vi "SubVI_Read_PHD_FromJSON_ver2.4.vi"(6 "Filter SIS by m/z?":bool, 7 "Nominal m/z for SIS hist finding\nComma separated":string, 8 "MAX Event Rate":dbl=0.1 format="%#_13g", 9 "MIN Event Rate":dbl=0.005 format="%#_13g", 10 "file (use dialog)":path) -> (1 "m/z in SIS Hist":dbl[](array[numeric]), 2 "Average SIS from Filtered Data":cluster{dbl[], dbl[]}(graph), 3 "Filtered SIS Hist in mV-ns":dbl[](array[numeric]), 5 "AverageSis":dbl)   [LabVIEW 2018]
uses:
  <vilib>/Analysis/baseanly.llb/Mean (DBL).vi
  <vilib>/Analysis/NI_AALPro.lvlib
  <vilib>/Analysis/NI_AALBase.lvlib
panel:
  out "min value":dbl
  out "SIS median":dbl format="%0.2f"
  out "SIS mean":dbl format="%0.2f"
  out "Original SIS Data":T1
  out "SpectrumCount":dbl
  out "User Filtered SIS Hist":T2(graph)
  out "Nbr Profiles":i32
  out "Profiles":T3(array[cluster])
  out "Original SIS Histogram":cluster{"Intensity":dbl[], "Frequency":dbl[]}(graph)
  out "JSON Text":string
  # "USER Filtering of SIS histogram data"
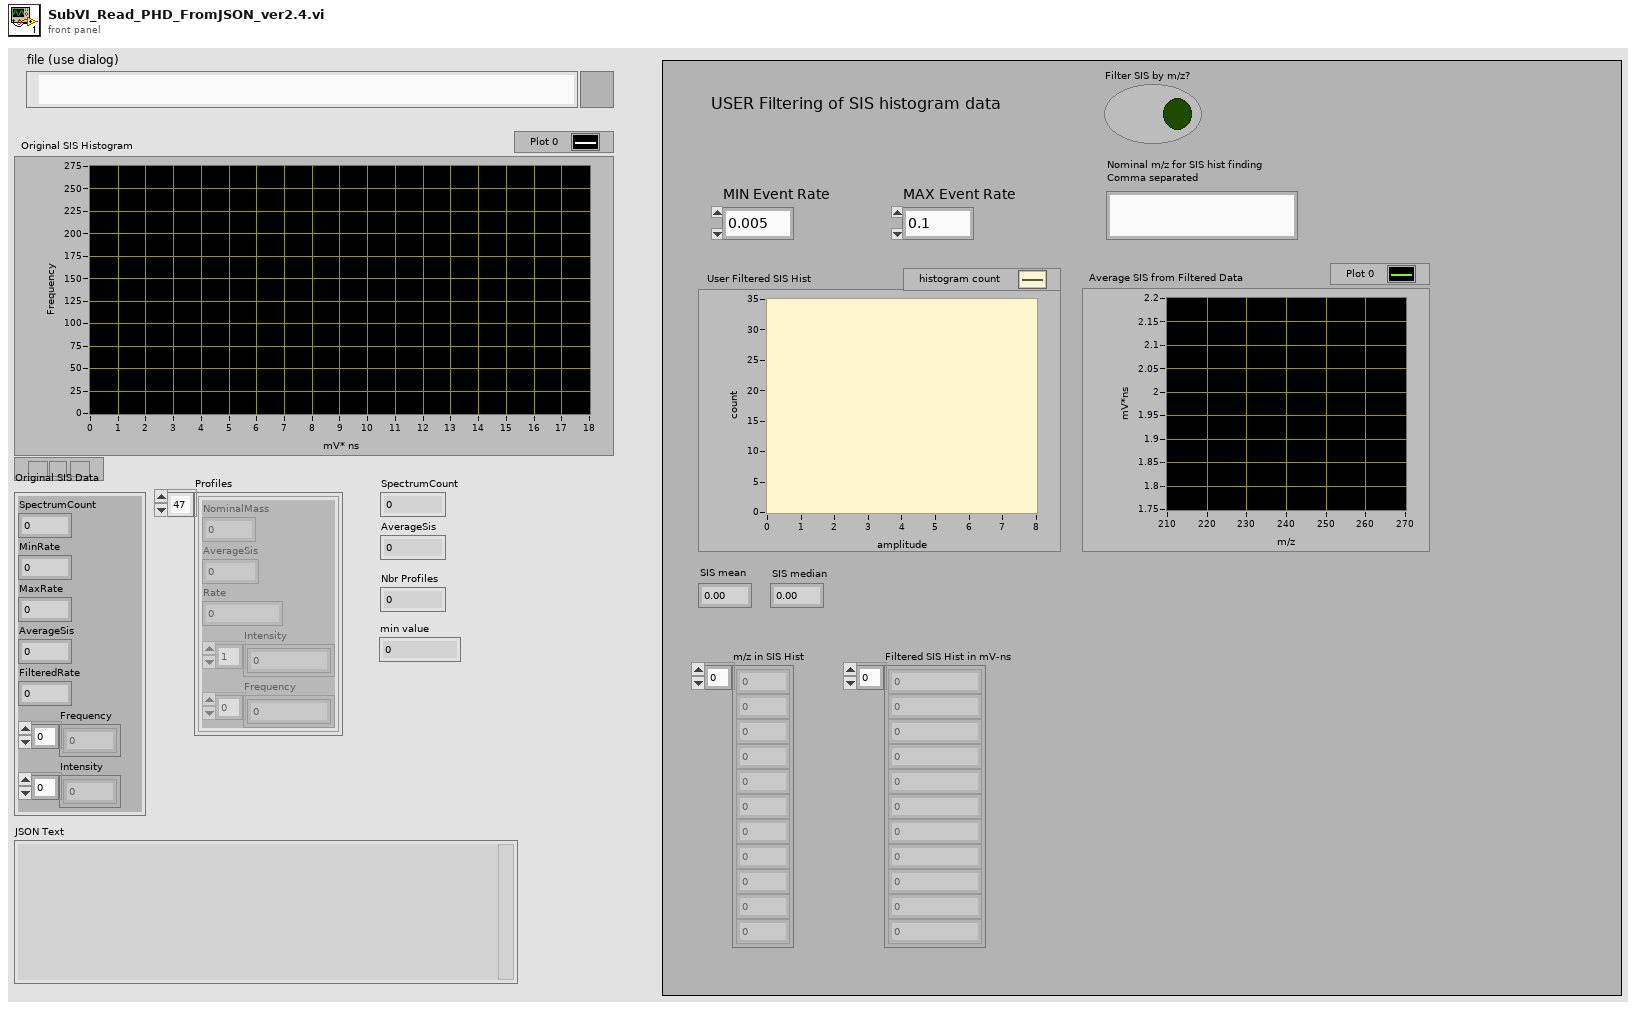
[diagram p1: front panel]
types:
  T1 = cluster{"SpectrumCount":dbl, "MinRate":dbl, "MaxRate":dbl, "AverageSis":dbl, "FilteredRate":dbl, "Frequency":dbl[], "Intensity":dbl[]}
  T2 = cluster{"X Values":dbl[], "Histogram: h(x)":i32[]}
  T3 = cluster{"NominalMass":dbl, "AverageSis":dbl, "Rate":dbl, "Intensity":dbl[], "Frequency":dbl[]}[]
  T4 = cluster{"Profiles":cluster{"NominalMass":dbl, "AverageSis":dbl, "Rate":dbl, "Intensity":dbl[], "Frequency":i32[]}[]}
  T5 = cluster{"NominalMass":dbl, "AverageSis":dbl, "Rate":dbl, "Intensity":dbl[], "Frequency":i32[]}[]
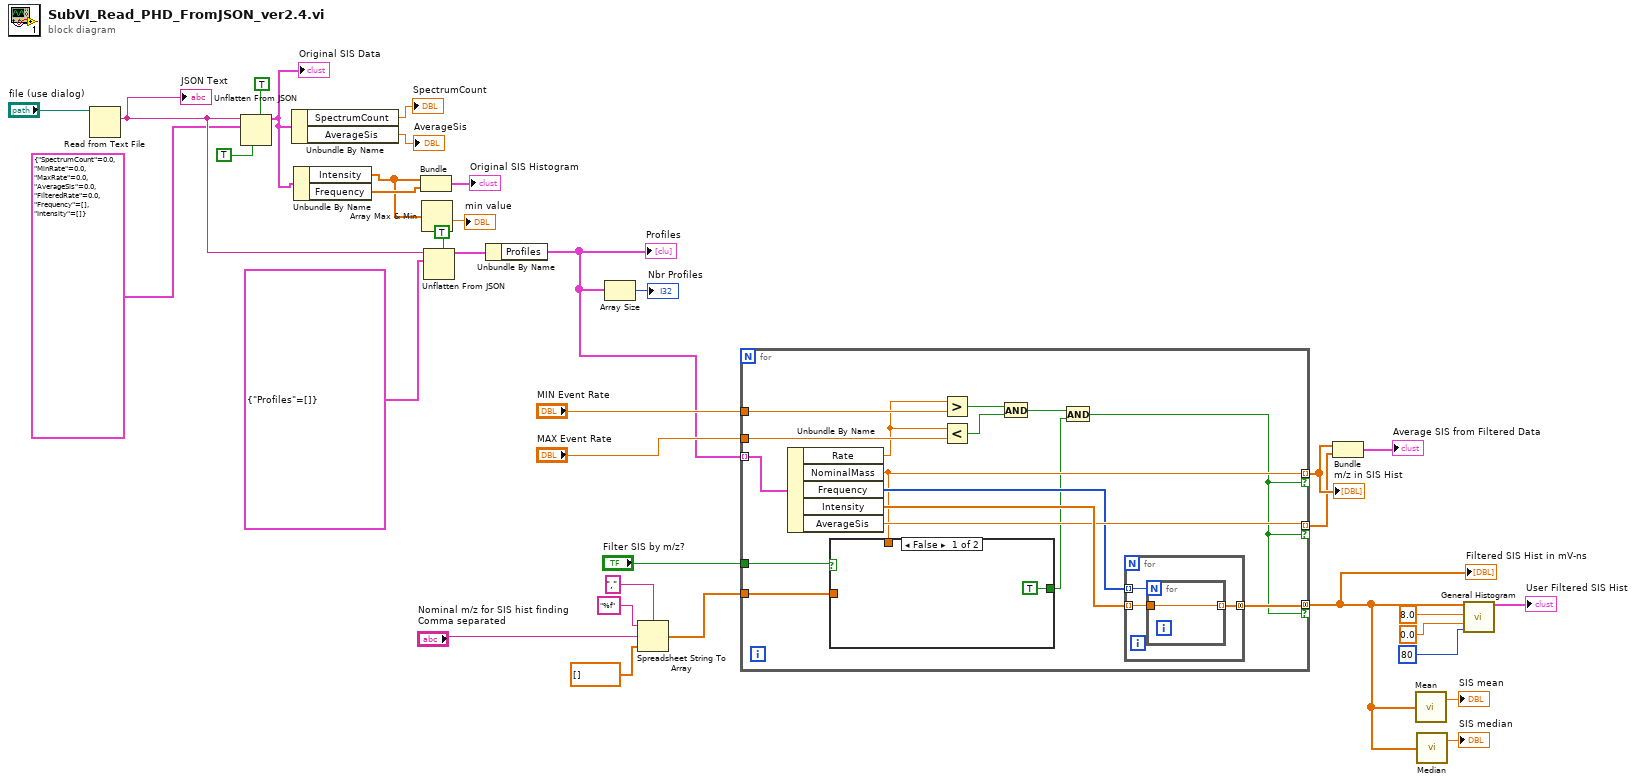
[diagram p0: block diagram]
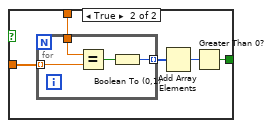
[diagram p2: hidden frame]
diagram:
  n1 = Read from Text File(file (use dialog)="file (use dialog)") -> (text=w31:string)  [unwired: 3 in, 3 out]
  "JSON Text" <- w31
  n2 = Unflatten From JSON(enable LabVIEW extensions? (T)=TRUE, JSON string=w31, type and defaults=T1 {"SpectrumCount"=0.0, "MinRate"=0.0, "MaxRate"=0.0, "AverageSis"=0.0, "FilteredRate"=0.0, "Frequency"=[], "Intensity"=[]}, default null elements? (F)=TRUE) -> (value=w24:T1)  [unwired: 3 in, 1 out]
  "Original SIS Data" <- w24
  n3 = Unbundle By Name(w24) -> ("SpectrumCount"=→"SpectrumCount":dbl, "AverageSis"=→"AverageSis":dbl)
  n4 = Unbundle By Name(w24) -> ("Intensity"=w1:dbl[], "Frequency"=w3:dbl[])
  n5 = Bundle("Intensity"=w1, "Frequency"=w3) -> (→"Original SIS Histogram":cluster{"Intensity":dbl[], "Frequency":dbl[]})  [unwired: 1 in]
  n6 = Array Max & Min(array=w1) -> (min value=→"min value":dbl)  [unwired: 3 out]
  n7 = Unflatten From JSON(enable LabVIEW extensions? (T)=TRUE, JSON string=w31, type and defaults=T4 {"Profiles"=[]}) -> (value=w28:T4)  [unwired: 4 in, 1 out]
  n8 = Unbundle By Name(w28) -> ("Profiles"=w17:T5)
  "Profiles" <- w17
  n9 = Array Size(array=w17) -> (size(s)=→"Nbr Profiles":i32)
  n10 = Spreadsheet String To Array(delimiter (Tab)=",", format string="%f", spreadsheet string="Nominal m/z for SIS hist finding\nComma separated", array type (2D Dbl)=dbl[] []) -> (array=w12:dbl[])
  n11 = for {
    tunnel: w17 -> [w51] mode=indexing
    tunnel: "MIN Event Rate" -> [w49]
    tunnel: "MAX Event Rate" -> [w48]
    tunnel: [w40] -> w6 mode=indexing if=w39
    tunnel: [w45] -> w8 mode=concatenating if=w39
    tunnel: [w44] -> w5 mode=indexing if=w39
    tunnel: w12 -> [w38]
    tunnel: "Filter SIS by m/z?" -> [w36]
    n12 = Unbundle By Name(w51) -> ("Rate"=w43:dbl, "NominalMass"=w40:dbl, "Frequency"=w42:i32[], "Intensity"=w46:dbl[], "AverageSis"=w44:dbl)
    n13 = case shown="False" w36 {
      tunnel: w40 -> [_ w57]
      tunnel: w38 -> [_ w56]
      tunnel: [TRUE w53] -> w37
      frame False {
      }
      frame True {
        n14 = for {
          tunnel: w57 -> [w61]
          tunnel: w56 -> [w60] mode=indexing
          tunnel: [w58] -> w55 mode=indexing
          n15 = Equal?(x=w61, y=w60) -> (x = y?=w59:bool)
          n16 = Boolean To (0,1)(Boolean=w59) -> (0, 1=w58:i16)
        }
        n17 = Add Array Elements(numeric array=w55) -> (sum=w54:i16)
        n18 = Greater Than 0?(x=w54) -> (x > 0?=w53:bool)
      }
    }
    n19 = Greater?(x=w43, y=w49) -> (0:w50:bool)
    n20 = Less?(x=w43, y=w48) -> (x < y?=w47:bool)
    n21 = And(x=w50, y=w47) -> (x .and. y?=w41:bool)
    n22 = And(x=w41, y=w37) -> (x .and. y?=w39:bool)
    n23 = for {
      tunnel: w42 -> [w62] mode=indexing
      tunnel: w46 -> [w64] mode=indexing
      tunnel: [w63] -> w45 mode=concatenating
      n24 = for {
        N: w62 -> [_]
        tunnel: w64 -> [w65]
        tunnel: [w65] -> w63 mode=indexing
      }
    }
  }
  "m/z in SIS Hist" <- w6
  "Filtered SIS Hist in mV-ns" <- w8
  n25 = Bundle(w6, w5) -> (→"Average SIS from Filtered Data":cluster{dbl[], dbl[]})  [unwired: 1 in]
  n26 = call-poly <vilib>:"Mean.vi"("X"=w8) -> ("mean"=→"SIS mean":dbl)  [unwired: 1 out]
  n27 = call <vilib>:"Median.vi"("X"=w8) -> ("median"=→"SIS median":dbl)  [unwired: 1 out]
  n28 = call <vilib>:"General Histogram.vi"("X"=w8, "max"=8.0, "min"=0.0, "# bins"=80) -> ("Histogram Graph"=→"User Filtered SIS Hist":T2)  [unwired: 7 in, 4 out]
